vi "format log entry.vi"(4 "error in (no error)":errorcluster, 5 "Username (\"\")":string, 6 "Module Name (\"\")":string, 7 "Error Type (Information)":T1) -> (0 "dup error in":errorcluster, 3 "Error Record":string)   [LabVIEW 2011]
uses:
  errorlog types.ctl
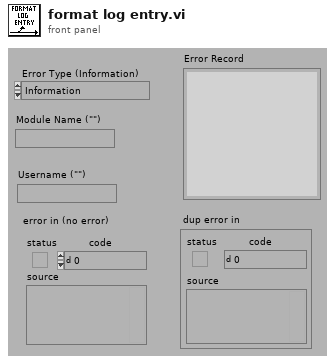
[diagram p1: front panel]
types:
  T1 = typedef "errorlog types.ctl" = enum16{"Information", "Warning", "Error"}
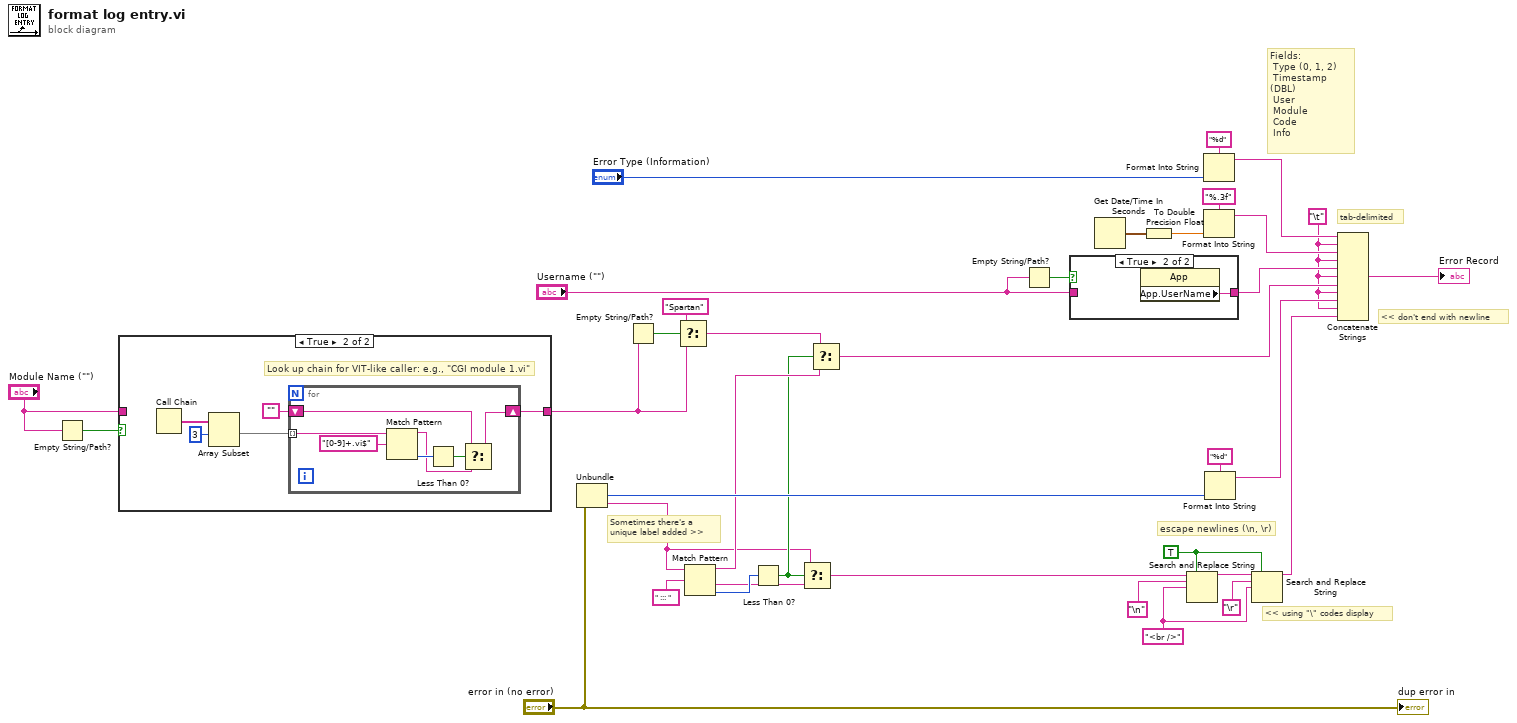
[diagram p0: block diagram]
diagram:
  w7 = "<br />" ("format string")
  w8 = TRUE
  w14 = "\t"
  # "Sometimes there's a\nunique label added >>"
  # "<< using \"\\\" codes display"
  # "escape newlines (\\n, \\r)"
  # "<< don't end with newline"
  # "tab-delimited"
  # "Fields:\n Type (0, 1, 2)\n Timestamp (DBL)\n User\n Module\n Code\n Info"
  n1 = Empty String/Path?(string/path="Module Name (\"\")") -> (empty?=w2:bool)
  n2 = case shown="True" w2 {
    tunnel: [w37 w41] -> w3
    tunnel: "Module Name (\"\")" -> [w37 _]
    frame False {
    }
    frame True {
      # "Look up chain for VIT-like caller: e.g., \"CGI module 1.vi\""
      n3 = Call Chain() -> (call chain=w40:string[])
      n4 = Array Subset(array=w40, index=3) -> (w38:string[])  [unwired: 1 in]
      n5 = for {
        shift-right: [w44] -> w41
        shift-left: "" -> [w45]
        tunnel: w38 -> [w48] mode=indexing
        n6 = Match Pattern(string=w48, regular expression="[0-9]+.vi$") -> (before substring=w43:string, offset past match=w47:i32)  [unwired: 3 out]
        n7 = Less Than 0?(x=w47) -> (x < 0?=w46:bool)
        n8 = Select(t=w45, s=w46, f=w43) -> (s? t:f=w44:string)
      }
    }
  }
  n9 = Unbundle("error in (no error)") -> ("code"=w35:i32, "source"=w29:string)  [unwired: 1 out]
  n10 = Empty String/Path?(string/path=w3) -> (empty?=w27:bool)
  n11 = Select(t="Spartan", s=w27, f=w3) -> (s? t:f=w5:string)
  n12 = Match Pattern(string=w29, regular expression=" ::: " ("format string")) -> (before substring=w32:string, after substring=w28:string, offset past match=w31:i32)  [unwired: 2 out]
  n13 = Less Than 0?(x=w31) -> (x < 0?=w30:bool)
  n14 = Select(t=w29, s=w30, f=w28) -> (s? t:f=w4:string)
  n15 = Select(t=w5, s=w30, f=w32) -> (s? t:f=w15:string)
  n16 = Empty String/Path?(string/path="Username (\"\")") -> (empty?=w24:bool)
  n17 = case shown="True" w24 {
    tunnel: [w50 w51] -> w17
    tunnel: "Username (\"\")" -> [w50 _]
    frame False {
    }
    frame True {
      n18 = property class="App"() -> ("App.UserName"=w51:string)  [unwired: 2 in, 2 out]
    }
  }
  n19 = Get Date/Time In Seconds() -> (seconds since 1Jan1904=w12:timestamp)
  n20 = To Double Precision Float(number=w12) -> (double precision float=w19:dbl)
  n21 = Search and Replace String(replace all?=w8, input string=w4, search string="\n" ("format string"), replace string=w7) -> (result string=w10:string)  [unwired: 1 in, 6 out]
  n22 = Format Into String(format string="%d", "Error Type (Information)") -> (resulting string=w21:string)  [unwired: 2 in, 1 out]
  n23 = Format Into String(format string="%.3f", w19) -> (resulting string=w18:string)  [unwired: 2 in, 1 out]
  n24 = Format Into String(format string="%d", w35) -> (resulting string=w16:string)  [unwired: 2 in, 1 out]
  n25 = Search and Replace String(replace all?=w8, input string=w10, search string="\r" ("format string"), replace string=w7) -> (result string=w9:string)  [unwired: 1 in, 6 out]
  n26 = Concatenate Strings(w21, w14, w18, w14, w17, w14, w15, w14, w16, w14, w9) -> (→"Error Record":string)
  "dup error in" <- "error in (no error)"
